vi "Volumetric Flow Rate Calculation.vi"() -> ()   [LabVIEW 2025]
uses:
  <vilib>/Utility/file.llb/Read Delimited Spreadsheet (string).vi
  <vilib>/Utility/file.llb/Read Delimited Spreadsheet (DBL).vi
panel:
  out "Differential Pressure":cluster{dbl[], dbl[]}(graph)
  in  "Psi":bool
  in  "Delay (ms)":dbl=0.1
  in  "Use spreadsheet?":bool
  out "XY Graph":cluster{"all rows":dbl[], dbl[]}(graph)
  in  "SpreadSheet 2":path
  out "max value":dbl
  in  "Tab Control":enum32{"Live Data", "Summary"}(tab)
  out "Thrust":dynamicdata(graph)
  out "Mass Flow Rate":dbl(graph)
  out "Upstream Pressure":dynamicdata(graph)
  out "Inlet Pressure":dynamicdata(graph)
  out "Differential Pressure 2":dynamicdata(graph)
  out "Supply Pressure":dynamicdata(graph)
  out "Chamber Pressure":dynamicdata(graph)
  out "Upstream \nTemperature":dynamicdata(graph)
  out "Inlet Temperature":dynamicdata(graph)
  out "Upstream Offset":dbl
  out "Inlet P. Offset":dbl
  out "Supply P. Offset":dbl
  out "Chamber Pressure":cluster{dbl[], dbl[]}[](graph)
  out "Supply Pressure":cluster{dbl[], dbl[]}(graph)
  out "Inlet Pressure":cluster{dbl[], dbl[]}(graph)
  out "Chamber Pressure":cluster{dbl[], dbl[]}(graph)
  out "Upstream Pressure 2":cluster{dbl[], dbl[]}(graph)
  out "Inlet Temp":cluster{dbl[], dbl[]}(graph)
  out "Upstream Temp":cluster{dbl[], dbl[]}(graph)
  out "Valve Position":cluster{dbl[], dbl[]}(graph)
  out "Thrust Profile":cluster{dbl[], dbl[]}(graph)
  out "Mass Flow Rate Plot":cluster{dbl[], dbl[]}(graph)
  out "Weight Scale":cluster{"all rows":dbl[], "all rows":dbl[]}(graph)
  in  "Boolean":bool
  in  "SpreadSheet":path
  out "Chamber P. Offset":dbl
  in  "Filename":path=path "C:/1. Rocket Research Project/CollectedData/Differential Pressure/0718_900PSI_Drain Tank.lvm"
  in  "stop":bool
  # "Choose a File to Analyze"
  # "Data Display"
  # "Pascal"
  # "Corrections"
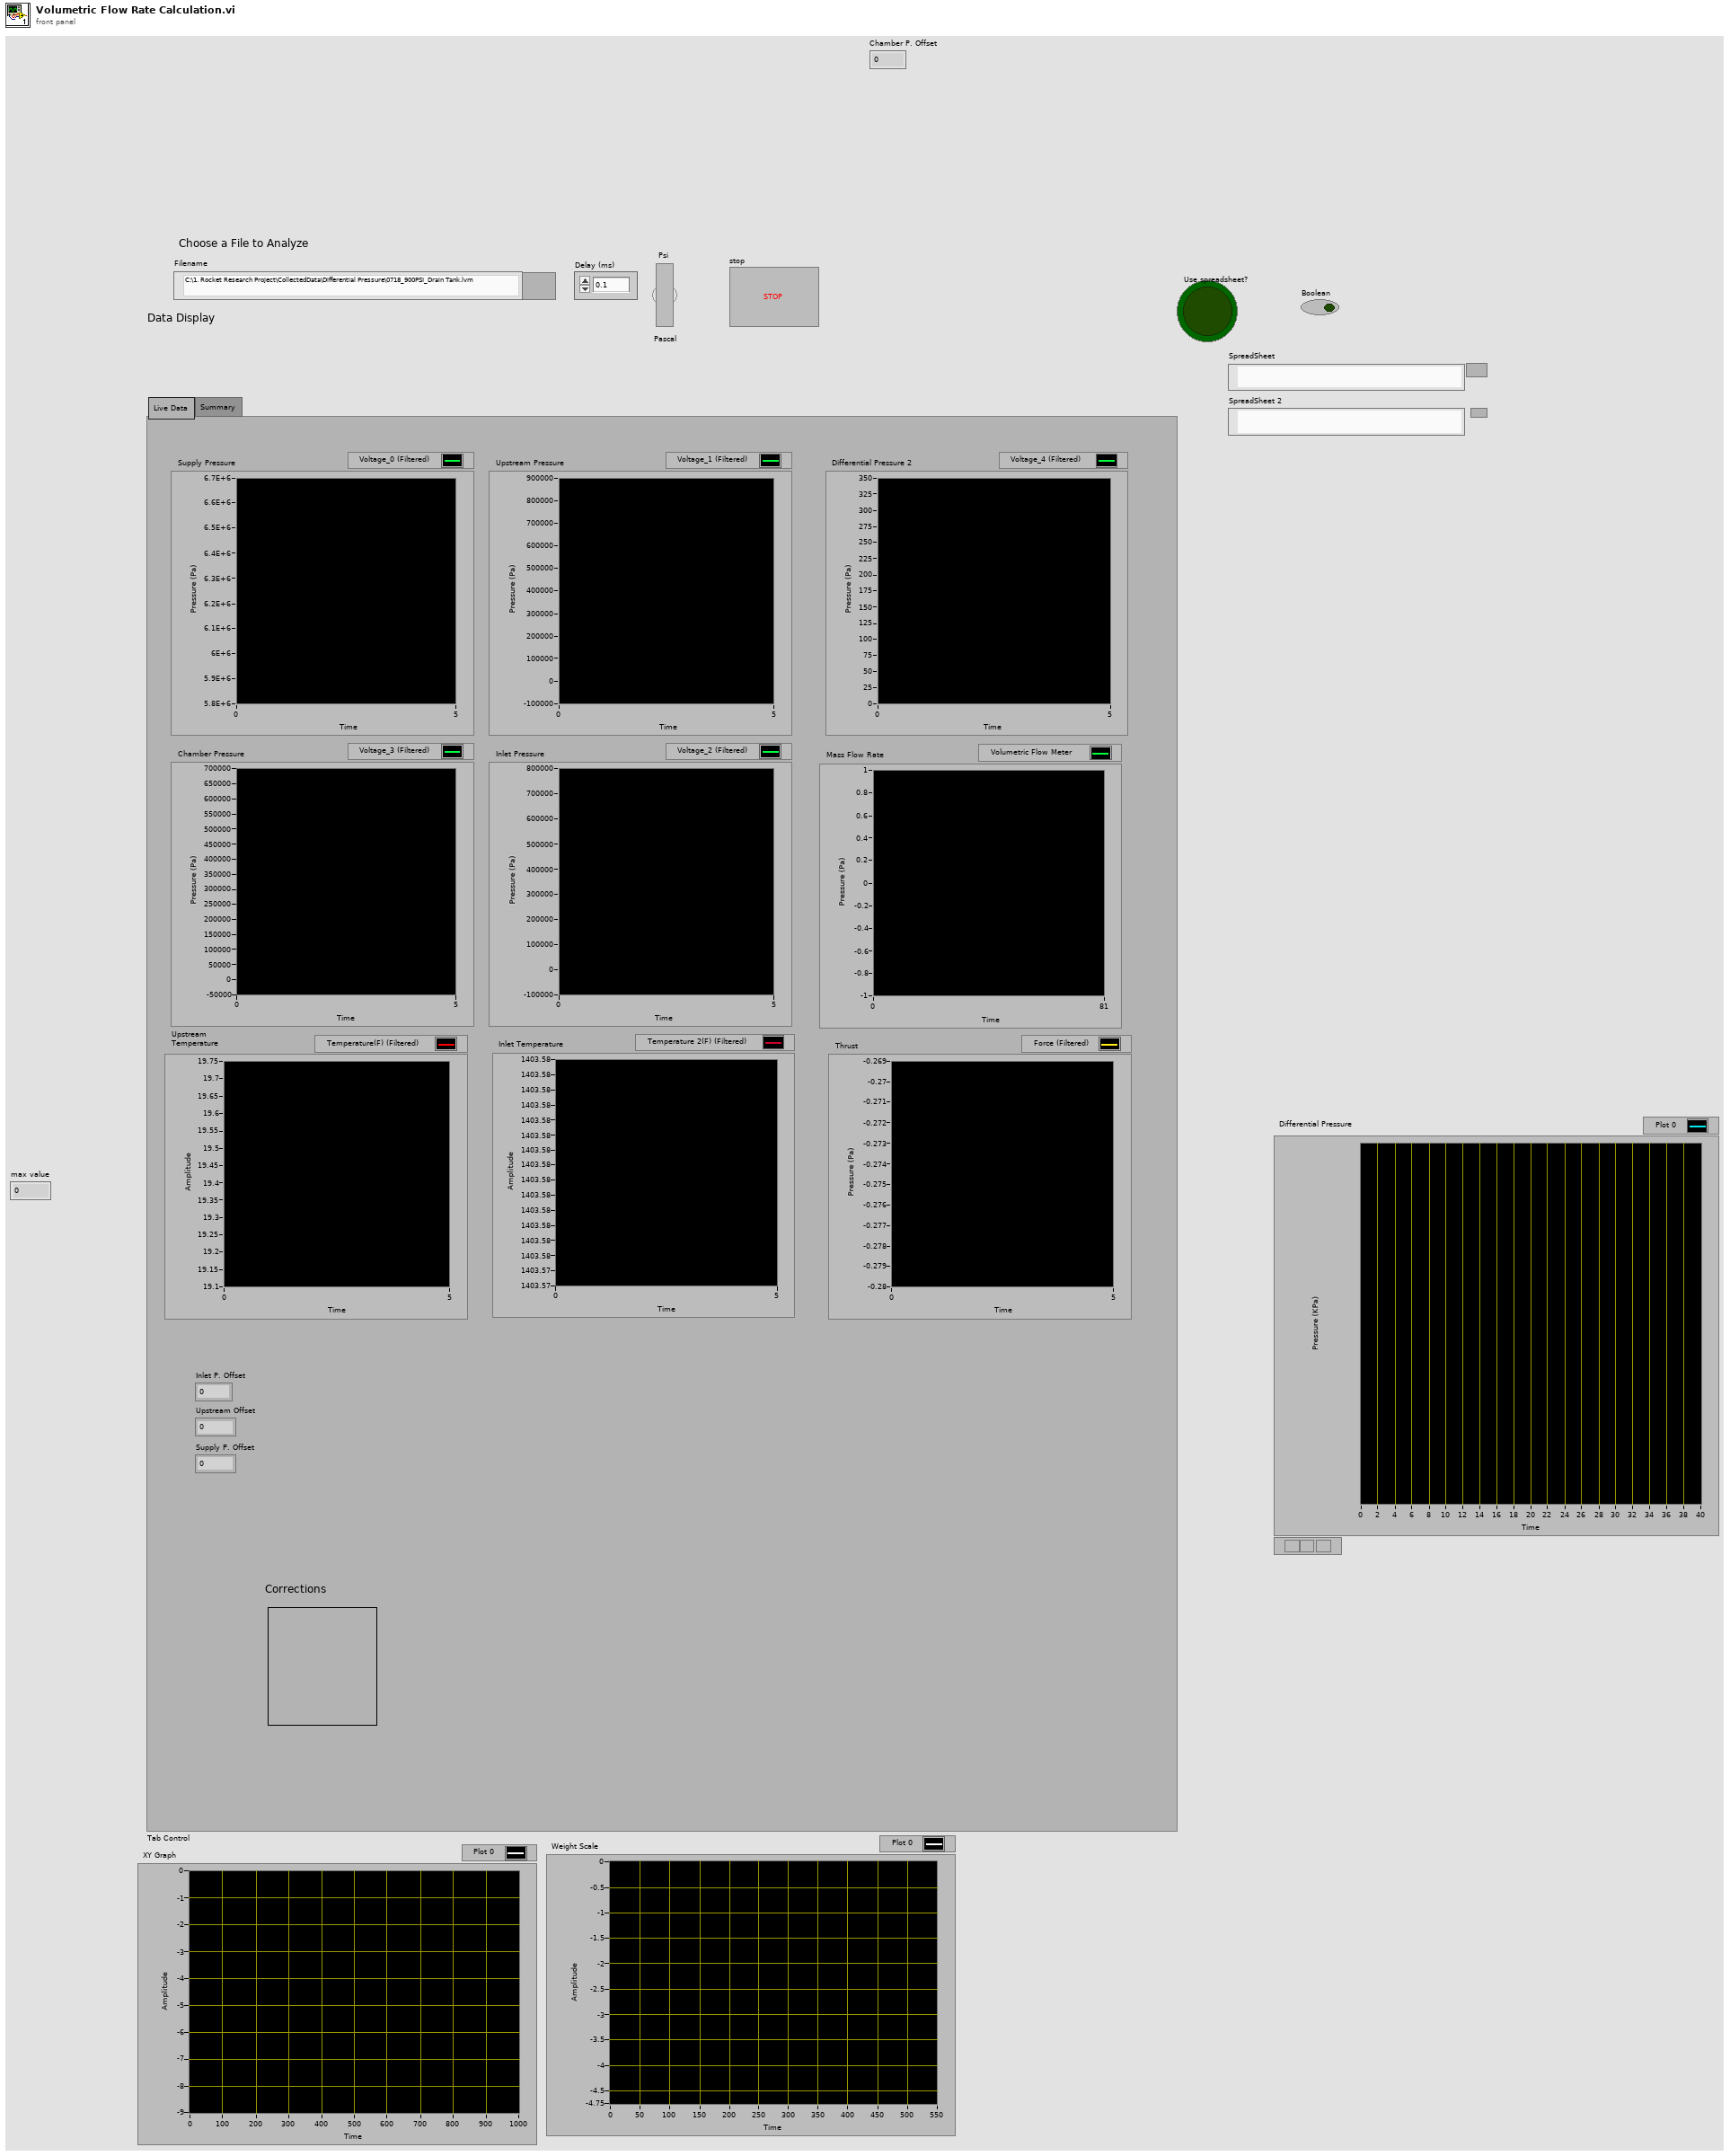
[diagram p1: front panel]
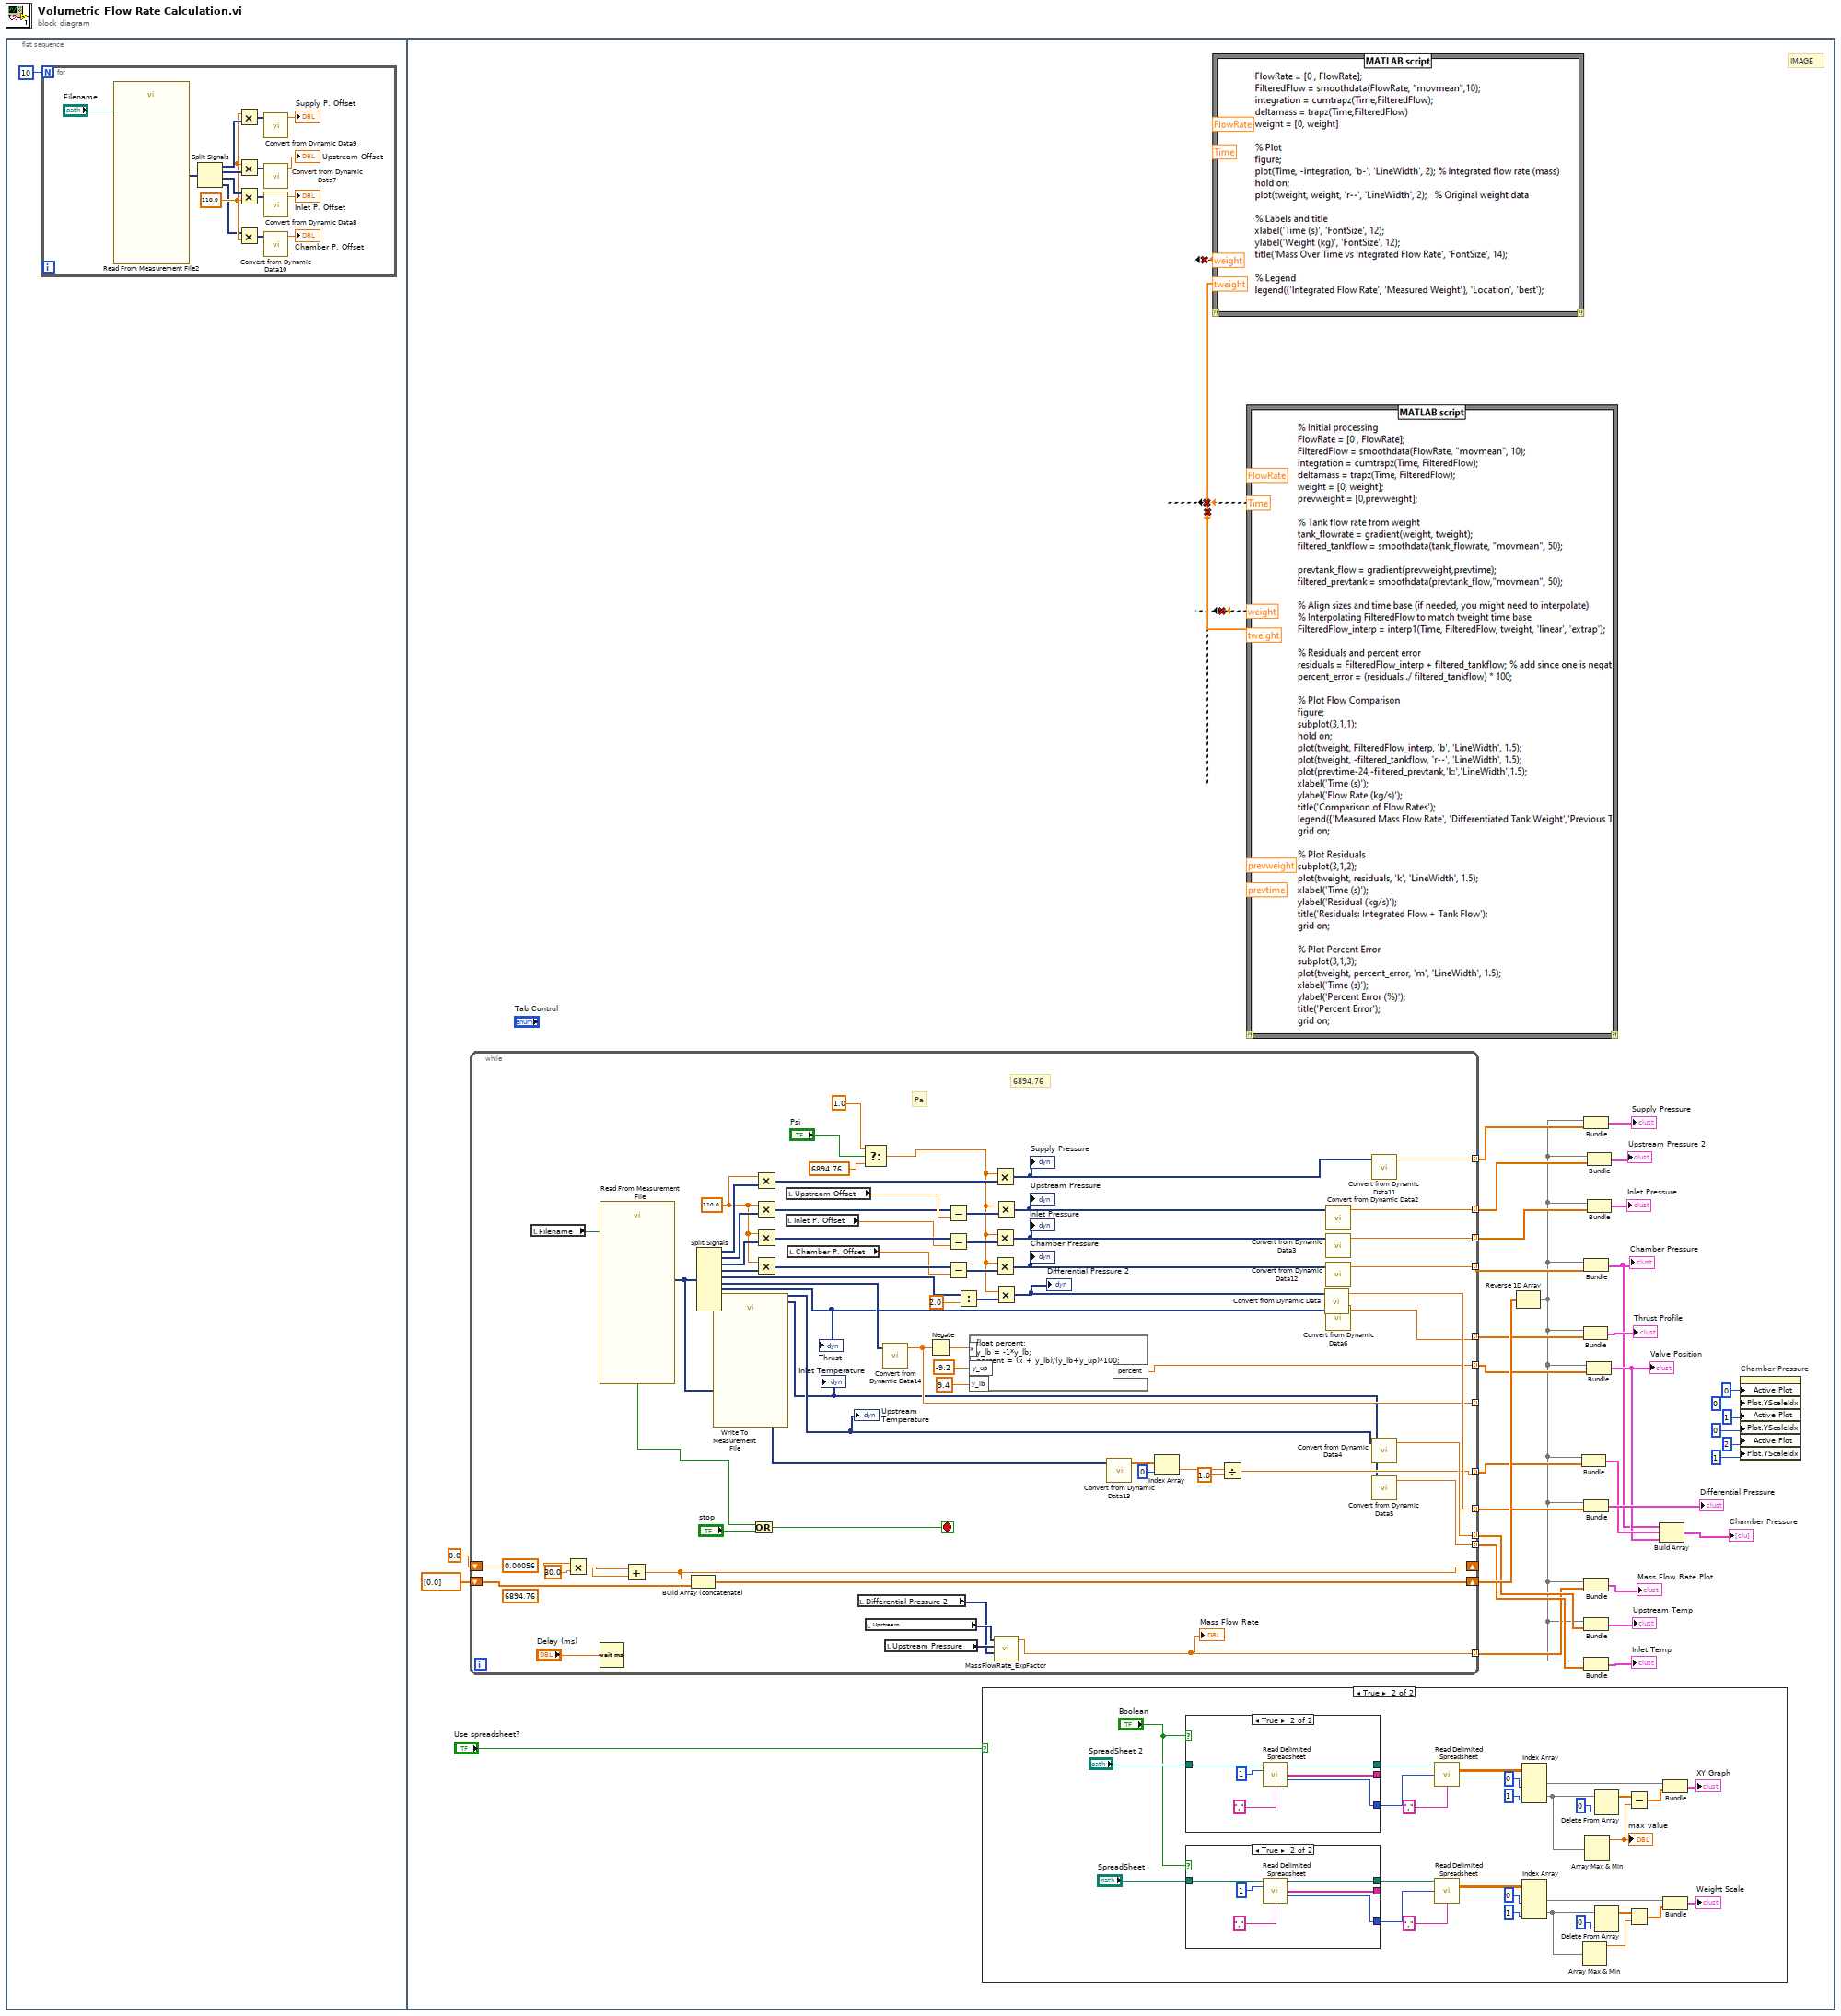
[diagram p0: block diagram]
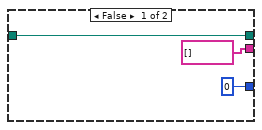
[diagram p3: hidden frame]
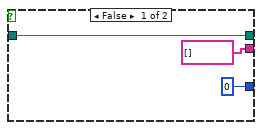
[diagram p4: hidden frame]
diagram:
  n1 = flat-sequence {
    frame #0 {
      n2 = for {
        N: 10 -> [_]
        w5 = 110.0 ("x")
        n3 = call "Read From Measurement File2"("Filename"="Filename") -> ("Signals"=w16:dynamicdata)  [unwired: 5 in, 5 out]
        n4 = Split Signals(w16) -> (w9:dynamicdata, w13:dynamicdata, w12:dynamicdata, w4:dynamicdata)  [unwired: 4 in]
        n5 = Multiply(x=w5, y=w9) -> (x*y=w8:dynamicdata)
        n6 = Multiply(x=w5, y=w13) -> (x*y=w14:dynamicdata)
        n7 = Multiply(x=w12, y=w5) -> (x*y=w11:dynamicdata)
        n8 = Multiply(x=w4, y=w5) -> (x*y=w3:dynamicdata)
        n9 = call "Convert from Dynamic Data9"("Dynamic Data Type"=w8) -> ("Scalar"=→"Supply P. Offset":dbl)  [unwired: 3 in]
        n10 = call "Convert from Dynamic Data7"("Dynamic Data Type"=w14) -> ("Scalar"=→"Upstream Offset":dbl)  [unwired: 3 in]
        n11 = call "Convert from Dynamic Data8"("Dynamic Data Type"=w11) -> ("Scalar"=→"Inlet P. Offset":dbl)  [unwired: 3 in]
        n12 = call "Convert from Dynamic Data10"("Dynamic Data Type"=w3) -> ("Scalar"=→"Chamber P. Offset":dbl)  [unwired: 3 in]
      }
    }
    frame #1 {
      # "IMAGE"
      n13 = while {
        shift-right: [w154] -> _
        shift-left: 0.0 -> [w157]
        shift-right: [w155] -> w48
        shift-left: dbl[] [0.0] -> [w156]
        tunnel: [w115] -> w44 mode=indexing
        tunnel: [w145] -> w42 mode=indexing
        tunnel: [w141] -> w39 mode=indexing
        tunnel: [w143] -> w37 mode=indexing
        tunnel: [w144] -> w36 mode=indexing
        tunnel: [w134] -> w22 mode=indexing
        tunnel: [w132] -> w46 mode=indexing
        tunnel: [w131] -> w45 mode=indexing
        tunnel: [w111] -> w24 mode=indexing
        tunnel: [w110] -> _ mode=indexing
        tunnel: [w106] -> w23 mode=indexing
        tunnel: [w103] -> w21 mode=indexing
        stop <- w163 stop-if-true
        (unwired) 6894.76 ("x")
        w138 = 110.0 ("x")
        # "6894.76"
        # "Pa"
        n14 = local read "Filename"() -> (w149:path)
        n15 = Multiply(x=0.00056, y=30.0) -> (x*y=w151:dbl)
        n16 = call "Read From Measurement File"("Filename"=w149) -> ("Signals"=w98:dynamicdata, "EOF?"=w162:bool)  [unwired: 5 in, 4 out]
        n17 = Wait (ms)(milliseconds to wait="Delay (ms)") -> ()  [unwired: 1 out]
        n18 = Add(x=w157, y=w151) -> (x+y=w154:dbl)
        n19 = Build Array (concatenate)(w154, w156) -> (w155:dbl[])
        n20 = Split Signals(w98) -> (w161:dynamicdata, w160:dynamicdata, w159:dynamicdata, w148:dynamicdata, w130:dynamicdata, w112:dynamicdata, w99:dynamicdata, w102:dynamicdata, w101:dynamicdata, w100:dynamicdata)  [unwired: 10 in]
        "Upstream \nTemperature" <- w102
        "Inlet Temperature" <- w101
        "Thrust" <- w99
        n21 = call "Write To Measurement File"("Signals"=w98) -> ()  [unwired: 16 in, 3 out]
        n22 = Or(x=w162, y="stop") -> (x .or. y?=w163:bool)
        n23 = Multiply(x=w138, y=w161) -> (x*y=w140:dynamicdata)
        n24 = Multiply(x=w138, y=w160) -> (x*y=w133:dynamicdata)
        n25 = Multiply(x=w138, y=w159) -> (x*y=w158:dynamicdata)
        n26 = Multiply(x=w138, y=w148) -> (x*y=w147:dynamicdata)
        n27 = local read "Inlet P. Offset"() -> (w150:dbl)
        n28 = local read "Upstream Offset"() -> (w139:dbl)
        n29 = local read "Chamber P. Offset"() -> (w146:dbl)
        n30 = local read "Differential Pressure 2"() -> (w116:dynamicdata)
        n31 = Select(t=1.0 ("f"), s="Psi", f=6894.76 ("t")) -> (s? t:f=w122:dbl)
        n32 = local read "Upstream \nTemperature"() -> (w118:dynamicdata)
        n33 = call "Convert from Dynamic Data14"("Dynamic Data Type"=w112) -> ("Scalar"=w110:dbl)  [unwired: 3 in]
        n34 = local read "Upstream Pressure"() -> (w117:dynamicdata)
        n35 = Negate(x=w110) -> (-x=w109:dbl)
        n36 = Subtract(x=w133, y=w139) -> (x-y=w136:dynamicdata)
        n37 = Subtract(x=w158, y=w150) -> (x-y=w137:dynamicdata)
        n38 = Subtract(x=w147, y=w146) -> (x-y=w135:dynamicdata)
        n39 = Divide(x=w130, y=2.0) -> (x/y=w126:dynamicdata)
        n40 = formula code="float percent;\ny_lb = -1*y_lb;\npercent = (x + y_lb)/(y_lb+y_up)*100;"("y_lb"=9.4 ("input variable"), "y_up"=-9.2 ("input variable"), "x"=w109) -> ("percent"=w111:dbl)
        n41 = Multiply(x=w122, y=w140) -> (x*y=w124:dynamicdata)
        "Supply Pressure" <- w124
        n42 = Multiply(x=w122, y=w137) -> (x*y=w125:dynamicdata)
        "Inlet Pressure" <- w125
        n43 = Multiply(x=w122, y=w135) -> (x*y=w123:dynamicdata)
        "Chamber Pressure" <- w123
        n44 = Multiply(x=w122, y=w136) -> (x*y=w128:dynamicdata)
        "Upstream Pressure" <- w128
        n45 = Multiply(x=w122, y=w126) -> (x*y=w129:dynamicdata)
        "Differential Pressure 2" <- w129
        n46 = call "MassFlowRate_ExpFactor.vi"("Differential Pressure"=w116, "Upstream Pressure"=w117, "Upstream \nTemperature"=w118) -> ("Mass Flow Rate"=w115:dbl)  [unwired: 8 in]
        "Mass Flow Rate" <- w115
        n47 = call "Convert from Dynamic Data13"("Dynamic Data Type"=w100) -> ("Array"=w108:dbl[])  [unwired: 3 in]
        n48 = Index Array(array=w108, index=0) -> (element=w105:dbl)
        n49 = Divide(x=w105, y=1.0) -> (x/y=w106:dbl)
        n50 = call "Convert from Dynamic Data"("Dynamic Data Type"=w129) -> ("Scalar"=w134:dbl)  [unwired: 3 in]
        n51 = call "Convert from Dynamic Data2"("Dynamic Data Type"=w128) -> ("Scalar"=w141:dbl)  [unwired: 3 in]
        n52 = call "Convert from Dynamic Data3"("Dynamic Data Type"=w125) -> ("Scalar"=w143:dbl)  [unwired: 3 in]
        n53 = call "Convert from Dynamic Data12"("Dynamic Data Type"=w123) -> ("Scalar"=w144:dbl)  [unwired: 3 in]
        n54 = call "Convert from Dynamic Data6"("Dynamic Data Type"=w99) -> ("Scalar"=w103:dbl)  [unwired: 3 in]
        n55 = call "Convert from Dynamic Data11"("Dynamic Data Type"=w124) -> ("Scalar"=w145:dbl)  [unwired: 3 in]
        n56 = call "Convert from Dynamic Data4"("Dynamic Data Type"=w102) -> ("Scalar"=w132:dbl)  [unwired: 3 in]
        n57 = call "Convert from Dynamic Data5"("Dynamic Data Type"=w101) -> ("Scalar"=w131:dbl)  [unwired: 3 in]
      }
      n58 = case shown="True" "Use spreadsheet?" {
        frame False {
        }
        frame True {
          n59 = case shown="True" "Boolean" {
            tunnel: [w82 w86] -> w64
            tunnel: "SpreadSheet 2" -> [w82 w85]
            tunnel: [string[] [] w84] -> _
            tunnel: [0 ("mark after read (chars.)") w83] -> w63
            frame False {
            }
            frame True {
              n60 = call-poly <vilib>:"Read Delimited Spreadsheet.vi"("file path (dialog if empty)"=w85, "number of rows (all:-1)"=1, "delimiter (\\t)"="," ("delimiter (\\t)")) -> ("new file path (Not A Path if cancelled)"=w86:path, "first row"=w84:string[], "mark after read (chars.)"=w83:i32)  [unwired: 7 in, 3 out]
            }
          }
          n61 = case shown="True" "Boolean" {
            tunnel: [w91 w95] -> w79
            tunnel: "SpreadSheet" -> [w91 w94]
            tunnel: [string[] [] w93] -> _
            tunnel: [0 ("mark after read (chars.)") w92] -> w77
            frame False {
            }
            frame True {
              n62 = call-poly <vilib>:"Read Delimited Spreadsheet.vi"("file path (dialog if empty)"=w94, "number of rows (all:-1)"=1, "delimiter (\\t)"="," ("delimiter (\\t)")) -> ("new file path (Not A Path if cancelled)"=w95:path, "first row"=w93:string[], "mark after read (chars.)"=w92:i32)  [unwired: 7 in, 3 out]
            }
          }
          n63 = call-poly <vilib>:"Read Delimited Spreadsheet.vi"("file path (dialog if empty)"=w64, "start of read offset (chars.:0)"=w63, "delimiter (\\t)"="," ("delimiter (\\t)")) -> ("all rows"=w62:dbl[][])  [unwired: 7 in, 5 out]
          n64 = call-poly <vilib>:"Read Delimited Spreadsheet.vi"("file path (dialog if empty)"=w79, "start of read offset (chars.:0)"=w77, "delimiter (\\t)"="," ("delimiter (\\t)")) -> ("all rows"=w75:dbl[][])  [unwired: 7 in, 5 out]
          n65 = Index Array(array=w62, index (col) #1=0 ("disabled index (col)"), index (col) #2=1 ("index (col)")) -> (element #1=w52:dbl[], element #2=w55:dbl[])  [unwired: 2 in]
          n66 = Index Array(array=w75, index (col) #1=0 ("disabled index (col)"), index (col) #2=1 ("index (col)")) -> (element #1=w67:dbl[], element #2=w70:dbl[])  [unwired: 2 in]
          n67 = Array Max & Min(array=w70) -> (max value=w69:dbl)  [unwired: 3 out]
          n68 = Array Max & Min(array=w55) -> (max value=w51:dbl)  [unwired: 3 out]
          "max value" <- w51
          n69 = Delete From Array(array=w55, index=0) -> (array with subset deleted=w58:dbl[])  [unwired: 1 in, 1 out]
          n70 = Delete From Array(array=w70, index=0) -> (array with subset deleted=w68:dbl[])  [unwired: 1 in, 1 out]
          n71 = Subtract(x=w58, y=w51) -> (x-y=w53:dbl[])
          n72 = Subtract(x=w68, y=w69) -> (x-y=w66:dbl[])
          n73 = Bundle("all rows"=w52, w53) -> (→"XY Graph":cluster{"all rows":dbl[], dbl[]})  [unwired: 1 in]
          n74 = Bundle("all rows"=w67, w66) -> (→"Weight Scale":cluster{"all rows":dbl[], dbl[]})  [unwired: 1 in]
        }
      }
      n75 = Reverse 1D Array(array=w48) -> (reversed array=w20:dbl[])
      n76 = Bundle(w20, w23) -> (w32:cluster{dbl[], dbl[]})  [unwired: 1 in]
      n77 = Bundle(w20, w21) -> (→"Thrust Profile":cluster{dbl[], dbl[]})  [unwired: 1 in]
      n78 = Bundle(w20, w42) -> (→"Supply Pressure":cluster{dbl[], dbl[]})  [unwired: 1 in]
      n79 = Bundle(w20, w36) -> (w18:cluster{dbl[], dbl[]})  [unwired: 1 in]
      "Chamber Pressure" <- w18
      n80 = Bundle(w20, w22) -> (→"Differential Pressure":cluster{dbl[], dbl[]})  [unwired: 1 in]
      n81 = Bundle(w20, w44) -> (→"Mass Flow Rate Plot":cluster{dbl[], dbl[]})  [unwired: 1 in]
      n82 = Bundle(w20, w46) -> (→"Upstream Temp":cluster{dbl[], dbl[]})  [unwired: 1 in]
      n83 = Bundle(w20, w45) -> (→"Inlet Temp":cluster{dbl[], dbl[]})  [unwired: 1 in]
      n84 = Bundle(w20, w24) -> (w29:cluster{dbl[], dbl[]})  [unwired: 1 in]
      "Valve Position" <- w29
      n85 = Bundle(w20, w39) -> (→"Upstream Pressure 2":cluster{dbl[], dbl[]})  [unwired: 1 in]
      n86 = Bundle(w20, w37) -> (→"Inlet Pressure":cluster{dbl[], dbl[]})  [unwired: 1 in]
      n87 = Build Array(w18, w32, w29) -> (→"Chamber Pressure":cluster{dbl[], dbl[]}[])
      n88 = property on="Chamber Pressure" class="XYGraph (strict)"("Active Plot"=u32 0, "Plot.YScaleIdx"=u32 0 ("Plot.Y Scale Index"), "Active Plot"=u32 1, "Plot.YScaleIdx"=u32 0 ("Plot.Y Scale Index"), "Active Plot"=u32 2, "Plot.YScaleIdx"=u32 1 ("Plot.Y Scale Index")) -> ()  [unwired: 2 in, 2 out]
    }
  }
